vi "PwF_ToF_RefNumRegistryGet.vi"(8 "error in (no error)":errorcluster, 10 "refnum name":string="My Gyro RefNum") -> (0 "error out":errorcluster, 3 "PwF ToF Ref":T1)   [LabVIEW 2018]
uses:
  ToF_TypeDef/PwF ToF Ref.ctl
  ToF_TypeDef/PwF ToF RangingMode.ctl
  <vilib>/Rock Robotics/WPI/Utilities/Refnum Registry Operation.ctl
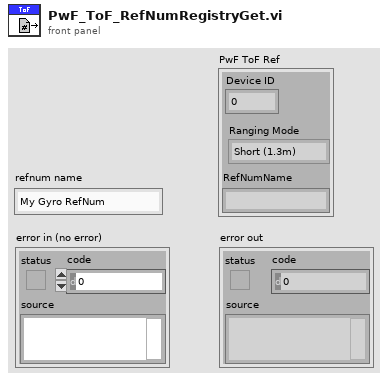
[diagram p1: front panel]
types:
  T1 = typedef "PwF ToF Ref.ctl" = cluster{"Device ID":u8, "Ranging Mode":T2, "RefNumName":string}
  T2 = typedef "PwF ToF RangingMode.ctl" = enum8{"Short (1.3m)", "Medium (2m)", "Long (4m)"}
  T3 = typedef "Refnum Registry Operation.ctl" = enum16{"set", "get", "delete", "get all names", "read name"}
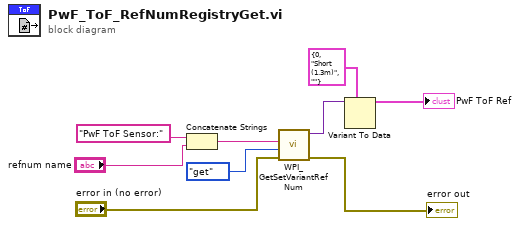
[diagram p0: block diagram]
diagram:
  n1 = Concatenate Strings("PwF ToF Sensor:", "refnum name") -> (w4:string)
  n2 = call <vilib>:"WPI_GetSetVariantRefNum.vi"("error in (no error)"="error in (no error)", "Operation"=Refnum_Registry_Operation."get", "refnum name"=w4) -> ("error out"=→"error out":errorcluster, "DevRef"=w9:variant)  [unwired: 6 in, 1 out]
  n3 = Variant To Data(type=T1 {"Device ID"=0, "Ranging Mode"=enum."Short (1.3m)", "RefNumName"=""}, Variant=w9) -> (data=→"PwF ToF Ref":T1)  [unwired: 1 in, 1 out]
